vi "Mutex Main.vi"() -> ()   [LabVIEW 2019]
uses:
  <vilib>/Platform/TimedLoop/XDataNode/timing_clust.ctl
  <vilib>/Platform/TimedLoop/XDataNode/nitl_modes.ctl
  <vilib>/Platform/TimedLoop/XDataNode/wakeup.ctl
  <vilib>/Platform/TimedLoop/XDataNode/loadnilvce.vi
  <vilib>/platform/TimedLoop/XDataNode/XDataNode.xnode
  <vilib>/Platform/TimedLoop/XDataNode/XDNodeRunTimeDep.lvlib
panel:
  out "TimeBtwEachItr (ms)":u32
  out "Status":T1
  out "Error":errorcluster
  in  "Stop":bool
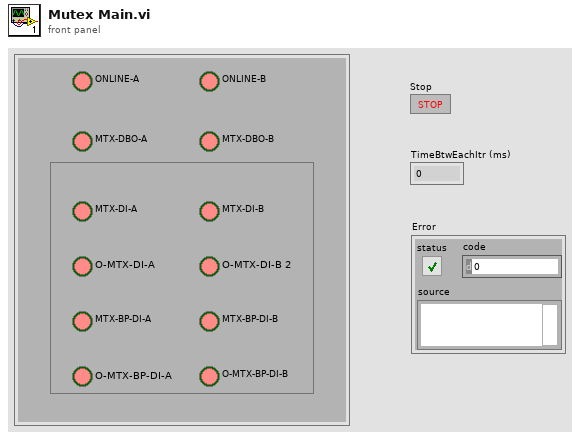
[diagram p1: front panel]
types:
  T1 = cluster{"MTX-DBO-A":bool, "ONLINE-A":bool, "Mutex Contacts":cluster{"MTX-DI-A":bool, "O-MTX-DI-A":bool, "MTX-BP-DI-A ":bool, "O-MTX-BP-DI-A":bool, "MTX-DI-B":bool, "O-MTX-DI-B 2":bool, "MTX-BP-DI-B":bool, "O-MTX-BP-DI-B":bool}, "MTX-DBO-B":bool, "ONLINE-B":bool}
  T2 = cluster{bool, bool, bool, bool, bool, bool, bool, bool}
  T3 = typedef "XDNodeRunTimeDep.lvlib/timing_clust.ctl" = cluster{"Expected End [f-1]":u64, "Actual End [f-1]":u64, "Finished Late? [f-1]":bool, "Expected End [i-1]":u64, "Actual End [i-1]":u64, "Finished Late? [i-1]":bool, "Expected Start [i]":u64, "Actual Start [i]":u64, "Expected Start [f]":u64, "Actual Start [f]":u64, "Source Name":string, "Structure Name":string, "Period":i64, "Deadline":i64, "Offset":i64, "Start":i64, "Priority":i32, "Timeout":i32, "Mode":T4, "Wakeup Reason":T5, "Error":errorcluster, "Source Type":string, "Secondary Source Type":string, "Global End Time":u64, "Global Start Time":u64, "Frame Duration":u64, "Iteration Duration":u64, "Assigned CPU":i32, "I/O Scan Engine Mode":u32}
  T4 = typedef "XDNodeRunTimeDep.lvlib/nitl_modes.ctl" = enum32{"No Change", "Process missed periods, maintain original phase", "Discard missed periods, maintain original phase", "Process missed periods, ignore original phase", "Discard missed periods, ignore original phase"}
  T5 = typedef "XDNodeRunTimeDep.lvlib/wakeup.ctl" = enum32{"Normal", "Aborted", "Asynchronous wakeup", "Timing source error", "Timed loop error", "Timeout"}
  T6 = cluster{bool, bool, cluster{bool, bool, bool, bool, bool, bool, bool, bool}, bool, bool}
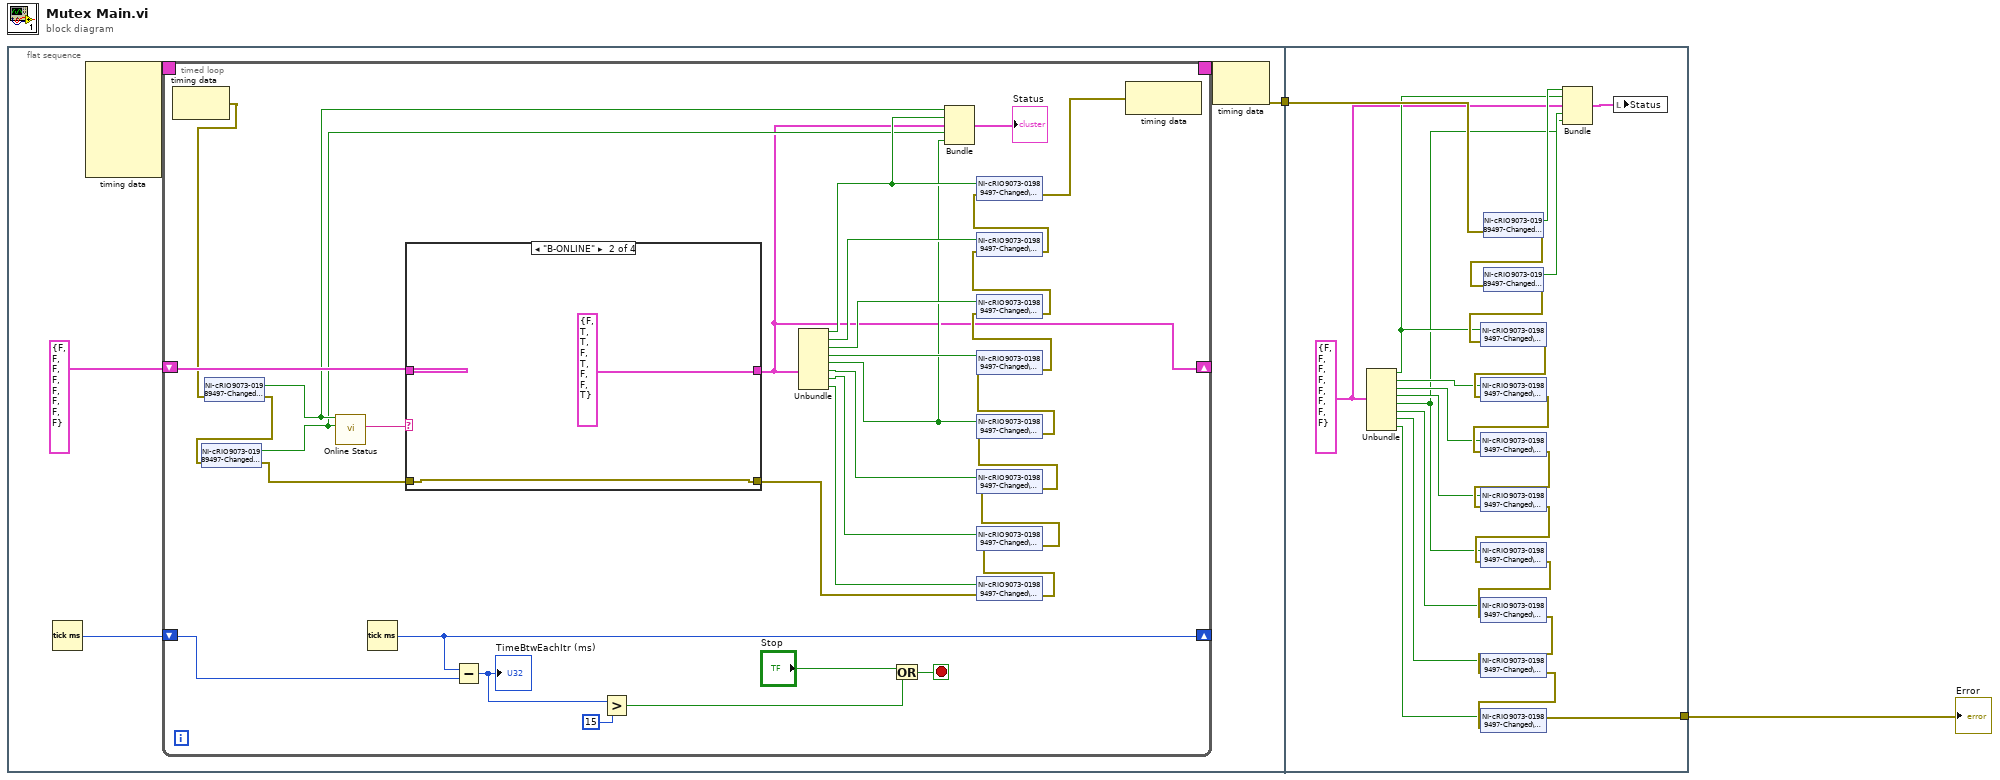
[diagram p0: block diagram]
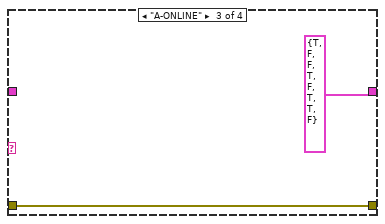
[diagram p3: hidden frame]
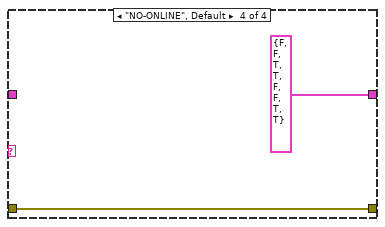
[diagram p4: hidden frame]
diagram:
  n1 = flat-sequence {
    tunnel: [w4] -> w2
    tunnel: [w78] -> w1
    tunnel: w2 -> [w69]
    frame #0 {
      n2 = Tick Count (ms)() -> (millisecond timer value=w3:u32)
      n3 = node-c288() -> (w7:T3)  [unwired: 6 in]
      n4 = timed-loop {
        timing: w7 -> [_]
        timing-out: [_] -> w6
        shift-right: [w16] -> _
        shift-left: T2 {FALSE, FALSE, FALSE, FALSE, FALSE, FALSE, FALSE, FALSE} -> [w25]
        shift-right: [w15] -> _
        shift-left: w3 -> [w14]
        stop <- w11 stop-if-true
        n5 = node-c288() -> (w8:errorcluster)  [unwired: 1 in]
        n6 = shared-variable "NI-cRIO9073-01989497-Changed\\Mod1\\DI0"(error in=w8) -> (w20:bool, error out=w40:errorcluster)
        n7 = shared-variable "NI-cRIO9073-01989497-Changed\\Mod1\\DI1"(error in=w40) -> (w19:bool, error out=w17:errorcluster)
        n8 = call "Online Status.vi"("MTX_DBO-B"=w19, "MTX-DBO-A"=w20) -> ("UNIT ONLINE"=w18:string)  [unwired: 8 in]
        n9 = Tick Count (ms)() -> (millisecond timer value=w15:u32)
        n10 = case shown="\"B-ONLINE\"" w18 {
          tunnel: w17 -> [w41 w43 w46 w47]
          tunnel: [w41 w43 w46 w47] -> w24
          tunnel: [w42 T2 {FALSE, TRUE, TRUE, FALSE, TRUE, FALSE, FALSE, TRUE} T2 {TRUE, FALSE, FALSE, TRUE, FALSE, TRUE, TRUE, FALSE} T2 {FALSE, FALSE, TRUE, TRUE, FALSE, FALSE, TRUE, TRUE}] -> w16
          tunnel: w25 -> [w42 _ _ _]
          frame "RETAIN" {
          }
          frame "B-ONLINE" {
          }
          frame "A-ONLINE" {
          }
          frame "NO-ONLINE", Default {
          }
        }
        n11 = Subtract(x=w15, y=w14) -> (x-y=w9:u32)
        "TimeBtwEachItr (ms)" <- w9
        n12 = Greater?(x=w9, y=u32 15 ("x")) -> (0:w13:bool)
        n13 = Unbundle(w16) -> (w23:bool, w31:bool, w30:bool, w29:bool, w22:bool, w28:bool, w27:bool, w26:bool)
        n14 = Or(x="Stop", y=w13) -> (x .or. y?=w11:bool)
        n15 = Bundle(w20, w23, w16, w19, w22) -> (→"Status":T6)  [unwired: 1 in]
        n16 = shared-variable "NI-cRIO9073-01989497-Changed\\Mod2\\DO7"(w26, error in=w24) -> (error out=w39:errorcluster)
        n17 = shared-variable "NI-cRIO9073-01989497-Changed\\Mod2\\DO6"(w27, error in=w39) -> (error out=w38:errorcluster)
        n18 = shared-variable "NI-cRIO9073-01989497-Changed\\Mod2\\DO5"(w28, error in=w38) -> (error out=w37:errorcluster)
        n19 = shared-variable "NI-cRIO9073-01989497-Changed\\Mod2\\DO4"(w22, error in=w37) -> (error out=w36:errorcluster)
        n20 = shared-variable "NI-cRIO9073-01989497-Changed\\Mod2\\DO3"(w29, error in=w36) -> (error out=w35:errorcluster)
        n21 = shared-variable "NI-cRIO9073-01989497-Changed\\Mod2\\DO2"(w30, error in=w35) -> (error out=w34:errorcluster)
        n22 = shared-variable "NI-cRIO9073-01989497-Changed\\Mod2\\DO1"(w31, error in=w34) -> (error out=w33:errorcluster)
        n23 = shared-variable "NI-cRIO9073-01989497-Changed\\Mod2\\DO0"(w23, error in=w33) -> (error out=w32:errorcluster)
        n24 = node-c288(w32) -> ()  [unwired: 1 out]
      }
      n25 = node-c288(w6) -> (w4:errorcluster)
    }
    frame #1 {
      w57 = T2 {FALSE, FALSE, FALSE, FALSE, FALSE, FALSE, FALSE, FALSE}
      n26 = Unbundle(w57) -> (w59:bool, w64:bool, w63:bool, w62:bool, w58:bool, w71:bool, w72:bool, w65:bool)
      n27 = shared-variable "NI-cRIO9073-01989497-Changed\\Mod1\\DI0"(error in=w69) -> (w61:bool, error out=w68:errorcluster)
      n28 = shared-variable "NI-cRIO9073-01989497-Changed\\Mod1\\DI1"(error in=w68) -> (w60:bool, error out=w67:errorcluster)
      n29 = shared-variable "NI-cRIO9073-01989497-Changed\\Mod2\\DO0"(w59, error in=w67) -> (error out=w79:errorcluster)
      n30 = shared-variable "NI-cRIO9073-01989497-Changed\\Mod2\\DO1"(w64, error in=w79) -> (error out=w77:errorcluster)
      n31 = shared-variable "NI-cRIO9073-01989497-Changed\\Mod2\\DO2"(w63, error in=w77) -> (error out=w76:errorcluster)
      n32 = shared-variable "NI-cRIO9073-01989497-Changed\\Mod2\\DO3"(w62, error in=w76) -> (error out=w66:errorcluster)
      n33 = shared-variable "NI-cRIO9073-01989497-Changed\\Mod2\\DO4"(w58, error in=w66) -> (error out=w75:errorcluster)
      n34 = shared-variable "NI-cRIO9073-01989497-Changed\\Mod2\\DO5"(w71, error in=w75) -> (error out=w74:errorcluster)
      n35 = shared-variable "NI-cRIO9073-01989497-Changed\\Mod2\\DO6"(w72, error in=w74) -> (error out=w73:errorcluster)
      n36 = shared-variable "NI-cRIO9073-01989497-Changed\\Mod2\\DO7"(w65, error in=w73) -> (error out=w78:errorcluster)
      n37 = Bundle(w61, w59, w57, w60, w58) -> (w70:T6)  [unwired: 1 in]
      n38 = local write "Status"(w70) -> ()
    }
  }
  "Error" <- w1
